vi "ARM - LOCK.vi"(8 "error in (no error)":errorcluster, 11 "STATE":enum16{"LOCK", "UNLOCK"}(ring)) -> (0 "error out":errorcluster)   [LabVIEW 2023]
uses:
  <vilib>/Rock Robotics/WPI/Solenoid/WPI_SolenoidValue.ctl
  Global INIT.vi
  <vilib>/Rock Robotics/WPI/Solenoid/WPI_SolenoidGetEnum.vi
  <vilib>/Rock Robotics/WPI/Solenoid/WPI_SolenoidSetEnum.vi
panel:
  out "Value":T1
  out "INTENT":string
  out "Installed?":bool
  out "description":string
  in  "SIDE":enum16{"LEFT", "RIGHT"}(ring)
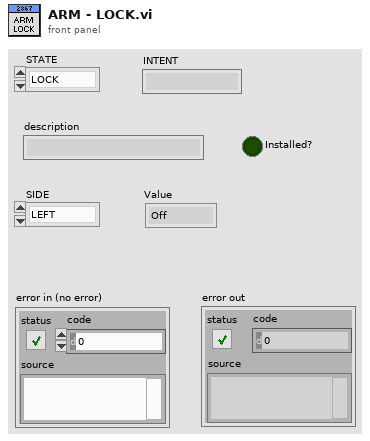
[diagram p1: front panel]
types:
  T1 = typedef "WPI_SolenoidValue.ctl" = enum16{"Off", "On", "Forward", "Reverse"}
  T2 = typedef "ctrl solenoid.ctl" = cluster{"description":string, "Installed?":bool, "refnum name":string, "coils":enum16{"Single", "Double"}, "forward channel":T3, "reverse channel":T3, "initial value":T1}
  T3 = typedef "WPI_SolenoidChannel.ctl" = enum8{"Solenoid 0", "Solenoid 1", "Solenoid 2", "Solenoid 3", "Solenoid 4", "Solenoid 5", "Solenoid 6", "Solenoid 7", "Solenoid 8", "Solenoid 9", "Solenoid 10", "Solenoid 11", "Solenoid 12", "Solenoid 13", "Solenoid 14", "Solenoid 15", "Invalid"}
  T4 = typedef "WPI_SolenoidDevRef.ctl" = cluster{"DevStatus":errorcluster, "Pneumatics Control Module":u8, "Forward Solenoid Channel":T3, "Reverse Solenoid Channel":T3}
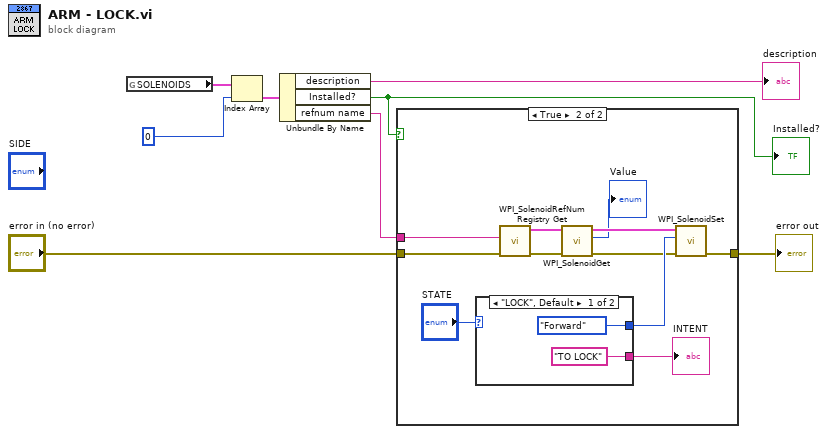
[diagram p0: block diagram]
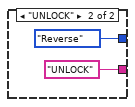
[diagram p3: hidden frame]
diagram:
  n1 = global read "Global INIT.vi" "SOLENOIDS"() -> (w8:T2[])
  n2 = Index Array(array=w8, index=0) -> (element=w7:T2)
  n3 = Unbundle By Name(w7) -> ("description"=→"description":string, "Installed?"=w5:bool, "refnum name"=w4:string)
  "Installed?" <- w5
  n4 = case shown="True" w5 {
    tunnel: w4 -> [_ w19]
    tunnel: "error in (no error)" -> [_ w15]
    tunnel: [_ w14] -> w3
    frame False {
    }
    frame True {
      n5 = case shown="\"LOCK\", Default" "STATE" {
        tunnel: [WPI_SolenoidValue."Forward" ("Value") WPI_SolenoidValue."Reverse" ("Value")] -> w16
        tunnel: ["TO LOCK" "UNLOCK"] -> w13
        frame "LOCK", Default {
        }
        frame "UNLOCK" {
        }
      }
      "INTENT" <- w13
      n6 = call <vilib>:"WPI_SolenoidRefNum Registry Get.vi"("error in (no error)"=w15, "refnum name"=w19) -> ("error out"=w11:errorcluster, "SolenoidDevRef"=w18:T4)  [unwired: 8 in]
      n7 = call-poly <vilib>:"WPI_SolenoidGet.vi"("error in (no error)"=w11, "SolenoidDevRef"=w18) -> ("error out"=w10:errorcluster, "Value"=→"Value":T1, "SolenoidDevRef"=w12:T4)  [unwired: 7 in]
      n8 = call-poly <vilib>:"WPI_SolenoidSet.vi"("error in (no error)"=w10, "Value"=w16, "SolenoidDevRef"=w12) -> ("error out"=w14:errorcluster)  [unwired: 7 in, 1 out]
    }
  }
  "error out" <- w3
